vi "Read Distance.vi"(8 "error in (no error)":errorcluster, 11 "Picture Ring in":refnum<class "Node.lvclass">) -> (0 "error out":errorcluster, 2 "Distance":i32, 3 "Picture Ring out":refnum<class "Node.lvclass">)   [LabVIEW 2019, in "Node.lvclass"]
uses:
  Node.lvclass
  Node.lvclass/Node.ctl
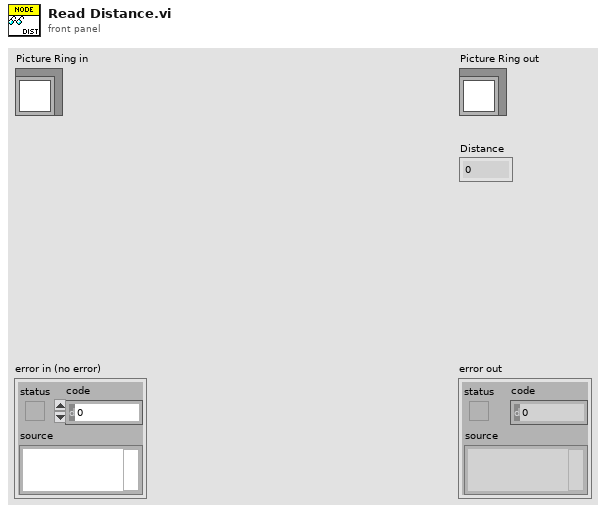
[diagram p1: front panel]
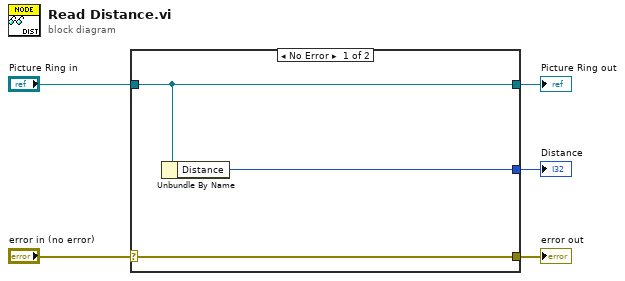
[diagram p0: block diagram]
diagram:
  n1 = case shown="No Error" "error in (no error)" {
    selector: "error in (no error)" -> [w8 w9]
    tunnel: [w8 w9] -> w4
    tunnel: [w7 w10] -> w2
    tunnel: "Picture Ring in" -> [w7 w10]
    tunnel: [w6 _] -> w1
    frame No Error {
      n2 = Unbundle By Name(w7) -> ("Distance"=w6:i32)
    }
    frame Error {
    }
  }
  "error out" <- w4
  "Picture Ring out" <- w2
  "Distance" <- w1
